vi "funcaoAvaliacaoGoleiroPrincipal.vi"(6 "Estado_Goleiro Atual":T1(ring), 8 "balls":T2[](array[typedef]), 9 "Robot in":T3, 11 "IA State":T8={"our_robots"=[], "enemy_robots"=[], "balls"=[], "geometry"={"field_length"=0, "field_width"=0, "goal_width"=0, "goal_depth"=0, "center_circle_radius"=0, "defense_width"=0, "defense_depth"=0, "free_kick_from_defense_dist"=0, "penalty_spot_from_field_line_dist"=0, "penalty_line_from_spot_dist"=0, "half_moon_depth"=0, "half_moon_width"=0}, "IA Judge"={"stage"="", "command"="", "our_goalie_id"=0.0, "enemy_goalie_id"=0.0, "command enum"=enum."Halt", "Time"=enum."Azul"}, "Received Timestamp"=timestamp(0 s since 1904-01-01), "Events"={"Touch"=FALSE, "id touch"=0.0, "Ball out of \nVision"=FALSE, "Ball inside \nGoalie area"=FALSE, "Robot not responding"=FALSE, "Robots responding status"=[1.0, 1.0, 1.0, 1.0, 1.0, 1.0], "Enemy Ball \nPossession"=FALSE, "Id ini Possession"=0.0, "Ball Possesion"=FALSE, "Id Possesion"=0.0, "Ball at\nour goal side"=FALSE, "Ball at\ntouchline"=FALSE, "Ball at\nenemy goal side"=FALSE}}) -> (3 "Estado_Goleiro":T1(ring))   [LabVIEW 2018]
uses:
  2019/VSS/Core/AI Input.ctl
  2019/VSS/Core/AI Robot.ctl
  2019/VSS/Intel/Functions Enum.ctl
  2019/VSS/Intel/AttackerStates.ctl
  2019/VSS/Path Planning/RRT/PathDests.ctl
  2019/VSS/Path Planning/RRT/PathDest.ctl
  2019/VSS/Core/AI Ball.ctl
  2019/VSS/Core/Field Size.ctl
  2019/VSS/Core/AI Judge.ctl
  2019/VSS/Intel/Command Enum.ctl
  2019/VSS/Util/Events/Events.ctl
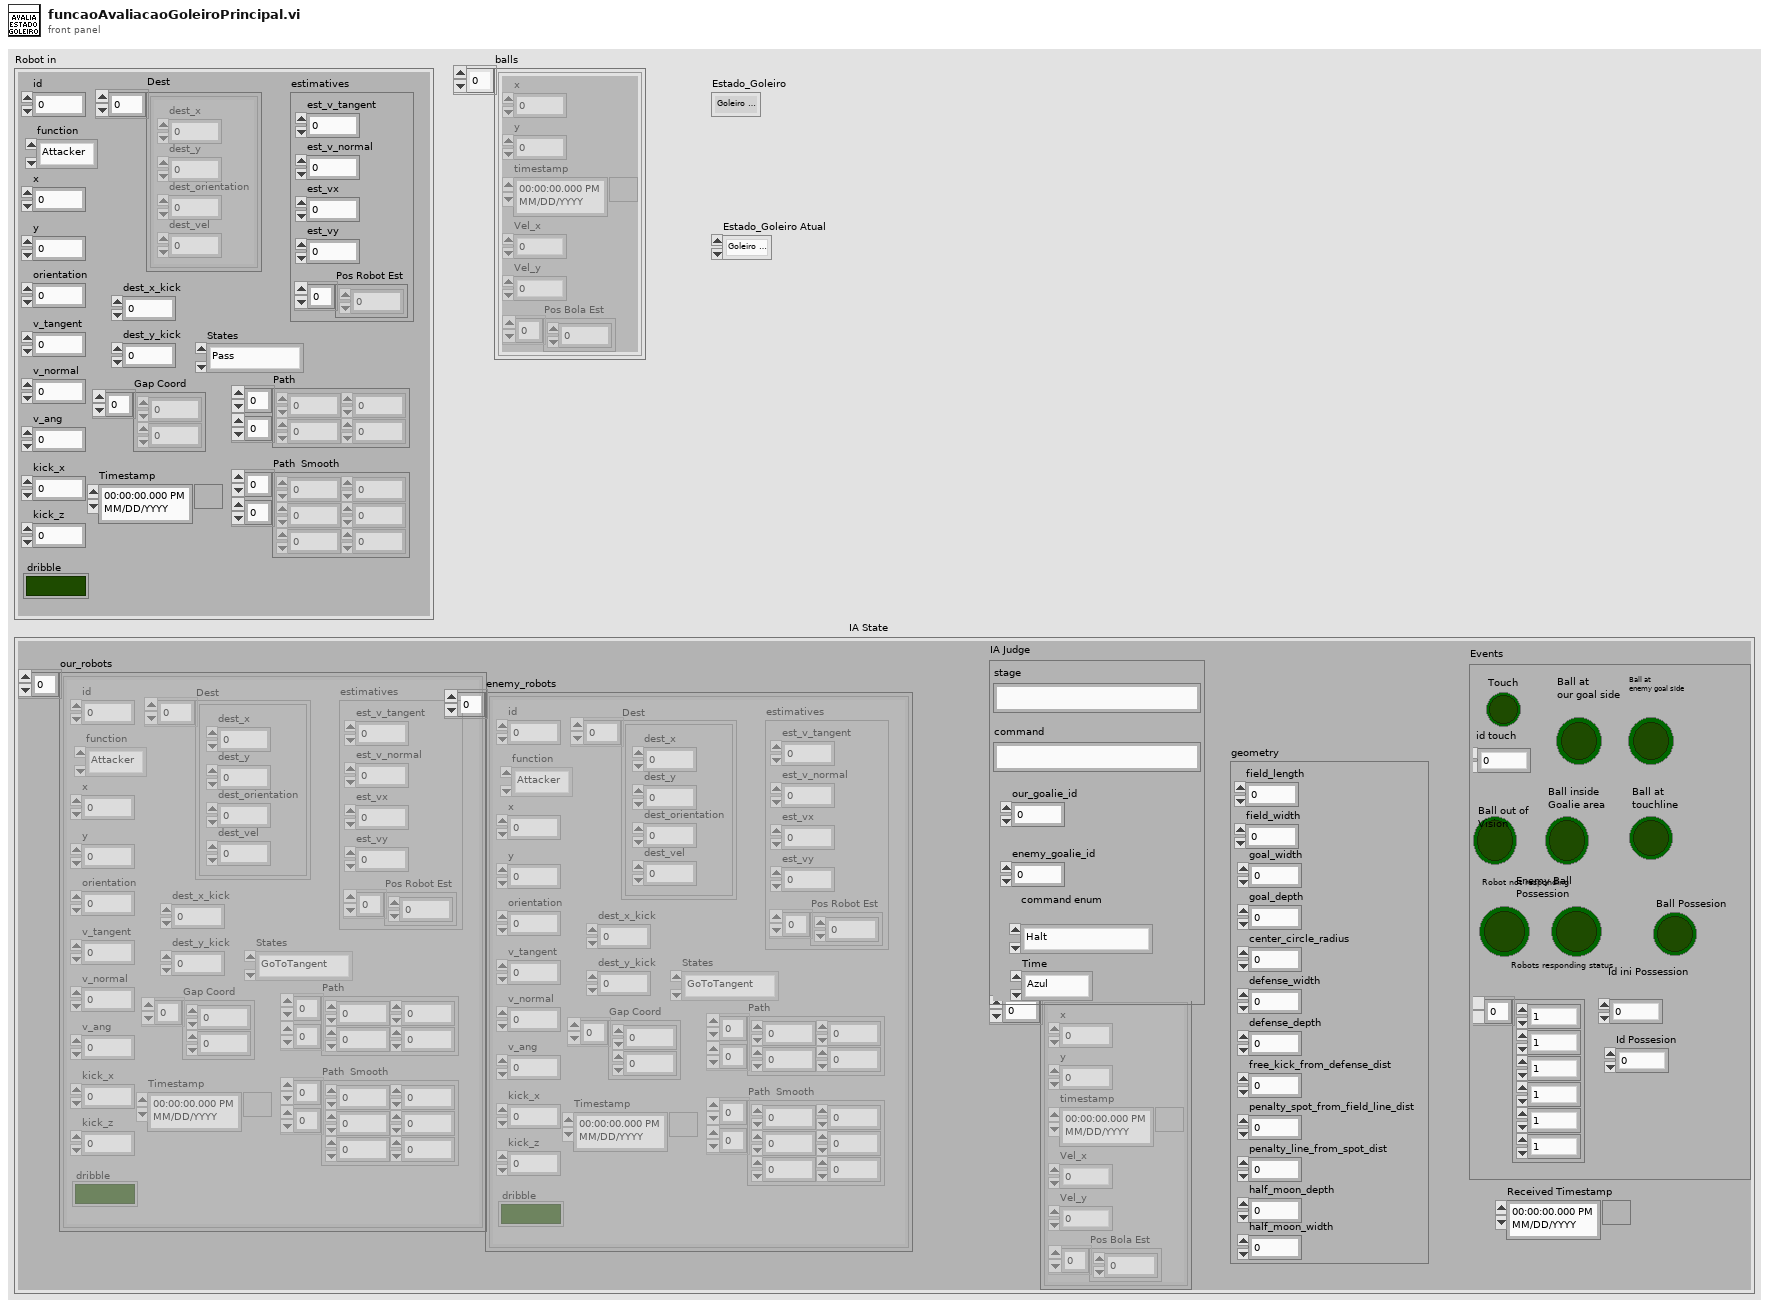
[diagram p1: front panel]
types:
  T1 = enum16{"Goleiro fora da área", "Alinhar com a bola", "Alinhar com a trave", "Rotacionar", "Aproximar-se da bola", "Posicionar-se na frente da bola"}
  T2 = typedef "AI Ball.ctl" = cluster{"x":dbl, "y":dbl, "timestamp":timestamp, "Vel_x":dbl, "Vel_y":dbl, "Pos Bola Est":dbl[]}
  T3 = typedef "AI Robot.ctl" = cluster{"id":u32, "function":T4, "x":dbl, "y":dbl, "orientation":dbl, "v_tangent":dbl, "v_normal":dbl, "v_ang":dbl, "kick_x":dbl, "kick_z":dbl, "dribble":bool, "Timestamp":timestamp, "estimatives":cluster{"est_v_tangent":dbl, "est_v_normal":dbl, "est_vx":dbl, "est_vy":dbl, "Pos Robot Est":dbl[]}, "dest_x_kick":dbl, "dest_y_kick":dbl, "Gap Coord":dbl[], "States":T5, "Path ":dbl[][], "Path  Smooth":dbl[][], "Dest":T6}
  T4 = typedef "Functions Enum.ctl" = enum16{"Attacker", "Goalie", "Defender", "Striker", "Goto 0", "Dummy", "Kicker", "ZigZag"}
  T5 = typedef "AttackerStates.ctl" = enum16{"Pass", "GoToTangent", "BallGetting", "GoToKick", "Rotate anti-clockwise", "Rotate Clockwise", ""}
  T6 = typedef "PathDests.ctl" = T7[]
  T7 = typedef "PathDest.ctl" = cluster{"dest_x":dbl, "dest_y":dbl, "dest_orientation":dbl, "dest_vel":dbl}
  T8 = typedef "AI Input.ctl" = cluster{"our_robots":T3[], "enemy_robots":T3[], "balls":T2[], "geometry":T9, "IA Judge":T10, "Received Timestamp":timestamp, "Events":T12}
  T9 = typedef "Field Size.ctl" = cluster{"field_length":u32, "field_width":u32, "goal_width":u32, "goal_depth":u32, "center_circle_radius":u32, "defense_width":u32, "defense_depth":u32, "free_kick_from_defense_dist":u32, "penalty_spot_from_field_line_dist":u32, "penalty_line_from_spot_dist":u32, "half_moon_depth":u32, "half_moon_width":u32}
  T10 = typedef "AI Judge.ctl" = cluster{"stage":string, "command":string, "our_goalie_id":dbl, "enemy_goalie_id":dbl, "command enum":T11, "Time":enum16{"Azul", "Amarelo"}}
  T11 = typedef "Command Enum.ctl" = enum16{"Halt", "Stop", "Force Start", "PKA Normal Start", "Prepare Kickoff Ally", "PKE Normal Start", "Prepare Kickoff Enemy", "Prepare Penalty Ally", "PPA Normal Start", "Prepare Penalty Enemy", "PPE Normal Start", "Ball Placement Enemy Up", "Ball Placement Enemy Down", "Ball Placement Ally Up", "Ball Placement Ally Mid", "Ball Placement Ally Down", "Indirect Free Enemy", "Indirect Free Ally", "Timeout Enemy", "Timeout Ally", "Goal Enemy", "Goal Ally", "Normal Half Time", "Extra Time Break", "Extra Half Time", "None", "Post Game"}
  T12 = typedef "Events.ctl" = cluster{"Touch":bool, "id touch":dbl, "Ball out of \nVision":bool, "Ball inside \nGoalie area":bool, "Robot not responding":bool, "Robots responding status":dbl[], "Enemy Ball \nPossession":bool, "Id ini Possession":dbl, "Ball Possesion":bool, "Id Possesion":dbl, "Ball at\nour goal side":bool, "Ball at\ntouchline":bool, "Ball at\nenemy goal side":bool}
  T13 = enum16{"Bola perto da area", "Bola longe da area"}
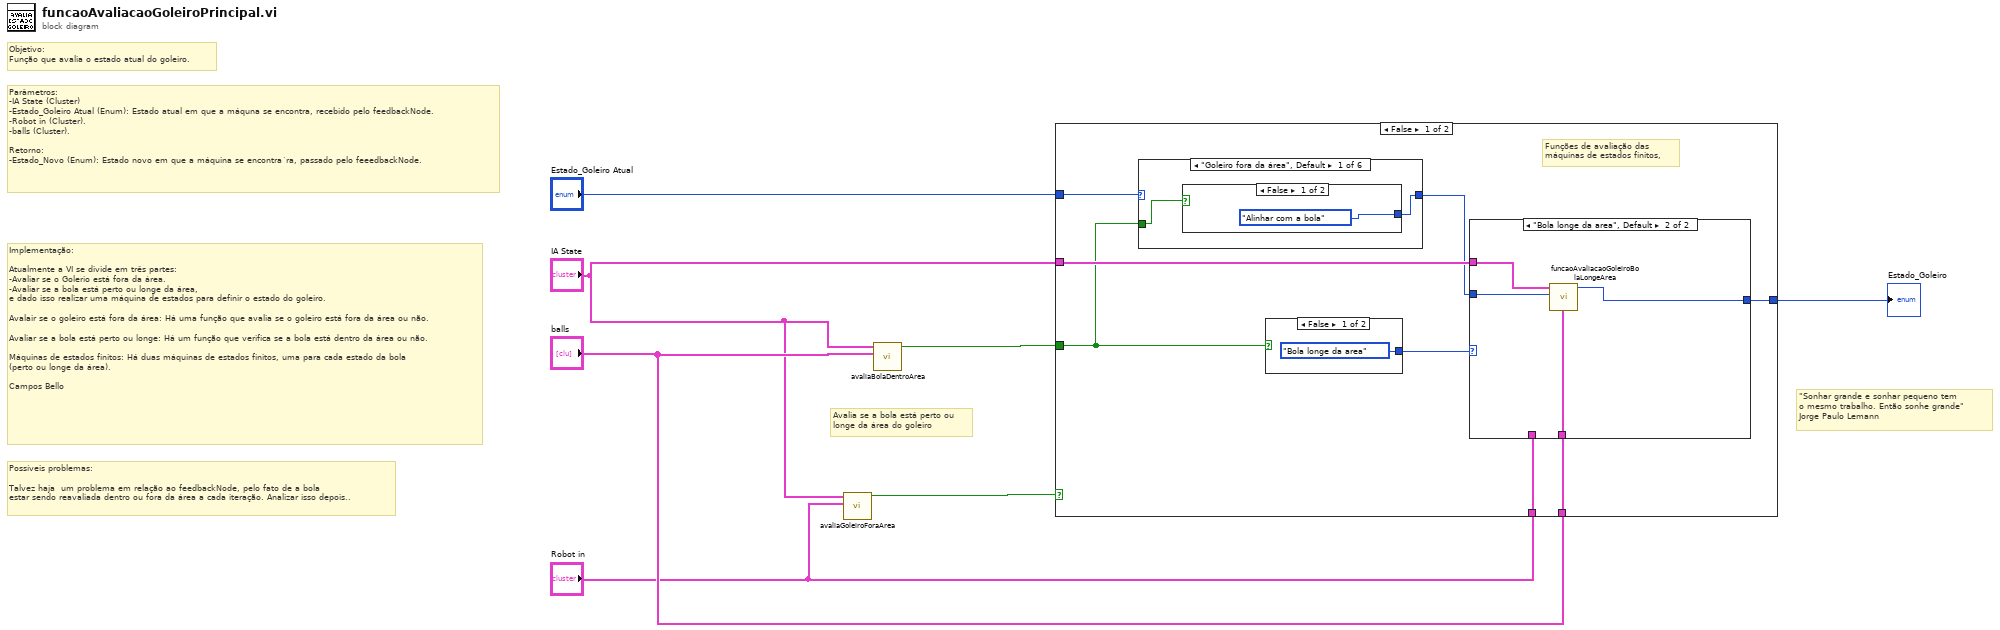
[diagram p0: block diagram]
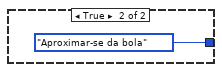
[diagram p2: hidden frame]
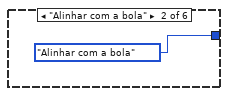
[diagram p3: hidden frame]
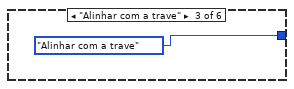
[diagram p4: hidden frame]
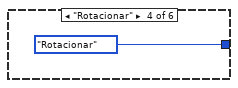
[diagram p5: hidden frame]
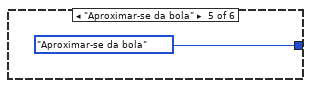
[diagram p6: hidden frame]
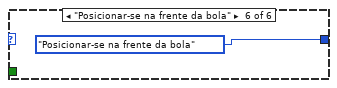
[diagram p7: hidden frame]
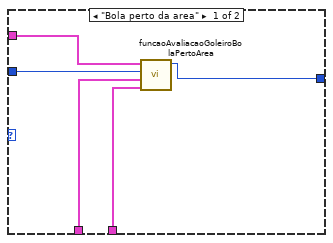
[diagram p8: hidden frame]
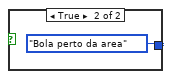
[diagram p9: hidden frame]
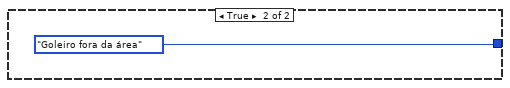
[diagram p10: hidden frame]
diagram:
  # "Avalia se a bola está perto ou \nlonge da área do goleiro"
  # "\"Sonhar grande e sonhar pequeno tem \no mesmo trabalho. Então sonhe grande\" \nJorge Paulo Lemann"
  # "Possíveis problemas:\n\nTalvez haja  um problema em relação ao feedbackNode, pelo fato de a bola\nestar sendo reavaliada dentro ou fora da área a cada iteração. Analizar isso depois.."
  # "Implementação:\n\nAtualmente a VI se divide em três partes: \n-Avaliar se o Golerio está fora da área.\n-Avaliar se a bola está perto ou longe da área, \ne dado isso realizar uma máquina de estados para definir o estado do goleiro.\n\nAvalair se o goleiro está fora da área: Há uma função que avalia se o goleiro está fora da área ou não.\n\nAvaliar se a bola está perto ou longe: Há um função que verifica se a bola está dentro da área ou não.\n\nMáquinas de estados finitos: Há duas máquinas de estados finitos, uma para cada estado da bola\n(perto ou longe da área).\n\nCampos Bello"
  # "Parâmetros:\n-IA State (Cluster)\n-Estado_Goleiro Atual (Enum): Estado atual em que a máquna se encontra, recebido pelo feedbackNode.\n-Robot in (Cluster).\n-balls (Cluster).\n\nRetorno:\n-Estado_Novo (Enum): Estado novo em que a máquina se encontra´ra, passado pelo feeedbackNode."
  # "Objetivo:\nFunção que avalia o estado atual do goleiro."
  n1 = call "avaliaGoleiroForaArea.vi"("Robot in"="Robot in", "IA State"="IA State") -> ("Goleiro fora da área?"=w1:bool)  [unwired: 9 in]
  n2 = call "avaliaBolaDentroArea.vi"("balls"="balls", "IA State"="IA State") -> ("Bola dentro da área"=w5:bool)  [unwired: 9 in]
  n3 = case shown="False" w1 {
    tunnel: [w14 T1."Goleiro fora da área" ("Estado_Goleiro")] -> w7
    tunnel: "balls" -> [w13 _]
    tunnel: w5 -> [w8 _]
    tunnel: "Estado_Goleiro Atual" -> [w9 _]
    tunnel: "IA State" -> [w12 _]
    tunnel: "Robot in" -> [w11 _]
    frame False {
      # "Funções de avaliação das \nmáquinas de estados finitos,"
      n4 = case shown="\"Goleiro fora da área\", Default" w9 {
        tunnel: [w16 T1."Alinhar com a bola" ("Estado_Goleiro Atual") T1."Alinhar com a trave" ("Estado_Goleiro Atual") T1."Rotacionar" ("Estado_Goleiro Atual") T1."Aproximar-se da bola" ("Estado_Goleiro Atual") T1."Posicionar-se na frente da bola" ("Estado_Goleiro Atual")] -> w10
        tunnel: w8 -> [w17 _ _ _ _ _]
        frame "Goleiro fora da área", Default {
          n5 = case shown="False" w17 {
            tunnel: [T1."Alinhar com a bola" ("Estado_Goleiro Atual") T1."Aproximar-se da bola" ("Estado_Goleiro Atual")] -> w16
            frame False {
            }
            frame True {
            }
          }
        }
        frame "Alinhar com a bola" {
        }
        frame "Alinhar com a trave" {
        }
        frame "Rotacionar" {
        }
        frame "Aproximar-se da bola" {
        }
        frame "Posicionar-se na frente da bola" {
        }
      }
      n6 = case shown="False" w8 {
        tunnel: [T13."Bola longe da area" ("Enum") T13."Bola perto da area" ("Enum")] -> w15
        frame False {
        }
        frame True {
        }
      }
      n7 = case shown="\"Bola longe da area\", Default" w15 {
        tunnel: w12 -> [w29 w33]
        tunnel: [w28 w32] -> w14
        tunnel: w11 -> [w27 _]
        tunnel: w13 -> [w26 w31]
        tunnel: w10 -> [w25 w30]
        frame "Bola perto da area" {
          n8 = call "funcaoAvaliacaoGoleiroBolaPertoArea.vi"("balls"=w26, "Robot in"=w27, "Estado_Atual"=w25, "IA State"=w29) -> ("Estado_Novo"=w28:T1)  [unwired: 7 in]
        }
        frame "Bola longe da area", Default {
          n9 = call "funcaoAvaliacaoGoleiroBolaLongeArea.vi"("balls"=w31, "Estado_Atual"=w30, "IA State"=w33) -> ("Estado_Novo"=w32:T1)  [unwired: 8 in]
        }
      }
    }
    frame True {
    }
  }
  "Estado_Goleiro" <- w7
